vi "OrderNotclose.vi"(8 "错误输入（无错误）":errorcluster, 9 "关闭通道":u16(ring) items=["CH1", "CH2", "CH3", "CH4"], 10 "打开通道":u16(ring) items=["CH1", "CH2", "CH3", "CH4"], 11 "VISA资源名称":refnum<visa-resource-name>="DPO5054-C012667") -> (0 "错误输出":errorcluster, 2 "输出数组":dbl[](array[numeric]), 3 "VISA资源名称 2":refnum<visa-resource-name>)   [LabVIEW 2014]
panel:
  out "AMP":dbl
  out "RMS":dbl
  out "MAX":dbl
  out "MIN":dbl
  out "PK2PK":dbl
  out "PERIOD":dbl
  out "FREQ":dbl
  out "RISETIME":dbl
  out "FallTime":dbl
  out "PosWidth":dbl
  out "NegWidth":dbl
  out "PositiveDutyCycle":dbl
  out "NegativeDutyCycle":dbl
  out "ACRMS":dbl
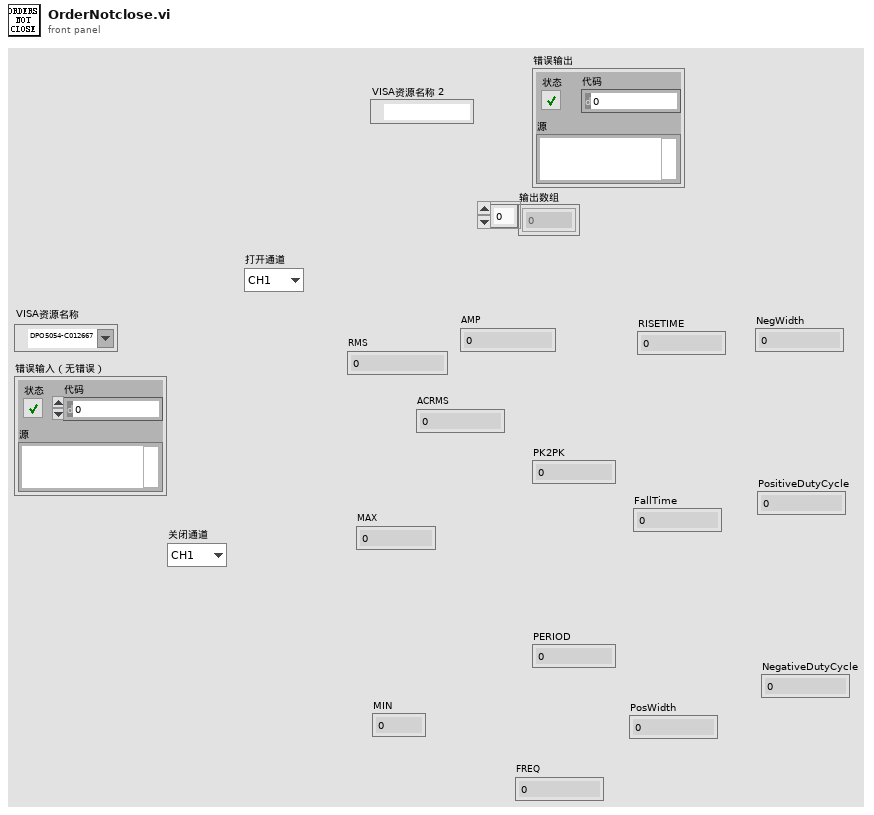
[diagram p1: front panel]
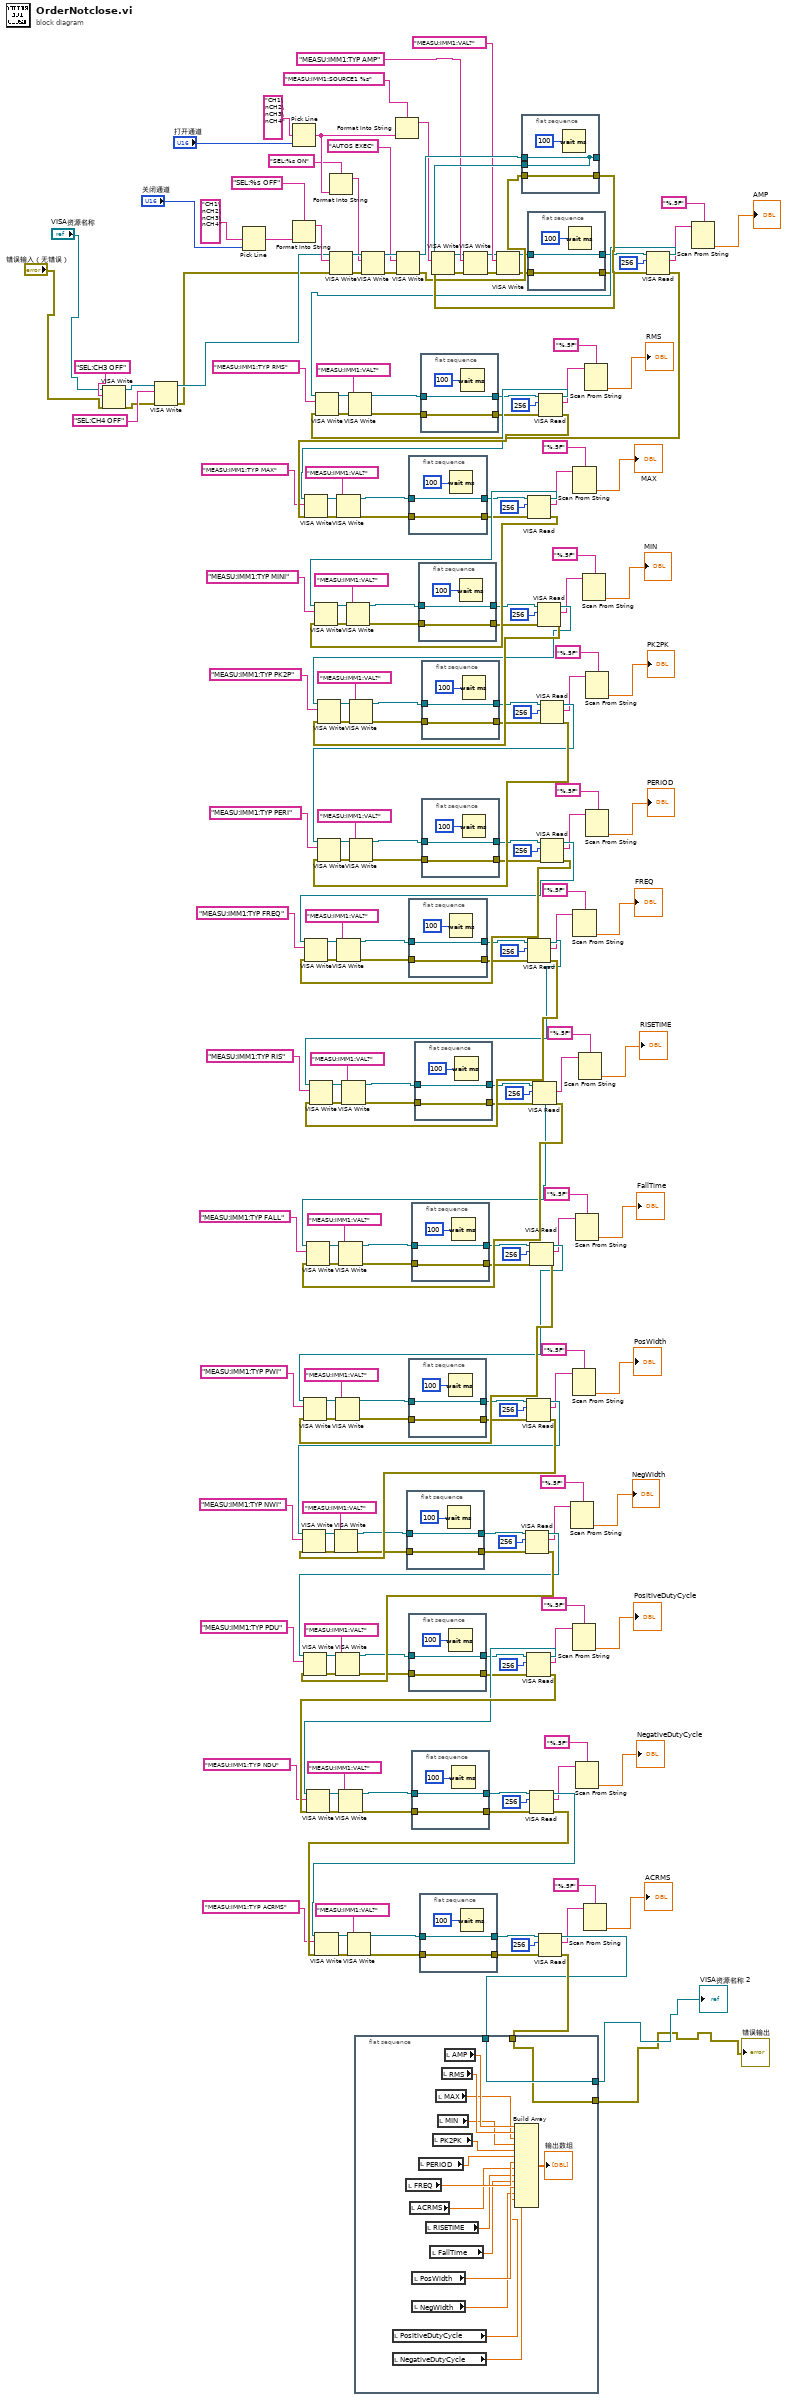
[diagram p0: block diagram]
diagram:
  n1 = VISA Write(VISA resource name="VISA资源名称", write buffer="SEL:CH3 OFF" ("格式字符串"), error in (no error)="错误输入（无错误）") -> (VISA resource name out=w6:refnum<visa-resource-name>, error out=w7:errorcluster)  [unwired: 1 out]
  n2 = VISA Write(VISA resource name=w6, write buffer="SEL:CH4 OFF" ("格式字符串"), error in (no error)=w7) -> (VISA resource name out=w2:refnum<visa-resource-name>, error out=w1:errorcluster)  [unwired: 1 out]
  n3 = Pick Line(multi-line string="CH1\nCH2\nCH3\nCH4" ("多行字符串"), line index="关闭通道") -> (output string=w30:string)  [unwired: 1 in]
  n4 = Pick Line(multi-line string="CH1\nCH2\nCH3\nCH4" ("多行字符串"), line index="打开通道") -> (output string=w25:string)  [unwired: 1 in]
  n5 = Format Into String(format string="SEL:%s OFF" ("格式字符串"), w30) -> (resulting string=w34:string)  [unwired: 2 in, 1 out]
  n6 = Format Into String(format string="SEL:%s ON" ("格式字符串"), w25) -> (resulting string=w26:string)  [unwired: 2 in, 1 out]
  n7 = VISA Write(VISA resource name=w2, write buffer=w34, error in (no error)=w1) -> (VISA resource name out=w35:refnum<visa-resource-name>, error out=w36:errorcluster)  [unwired: 1 out]
  n8 = flat-sequence {
    tunnel: w227 -> [w231]
    tunnel: [w231] -> w229
    tunnel: w228 -> [w230]
    tunnel: [w230] -> w9
    frame #0 {
      n9 = local read "PositiveDutyCycle"() -> (w234:dbl)
      n10 = local read "NegativeDutyCycle"() -> (w233:dbl)
      n11 = local read "FREQ"() -> (w240:dbl)
      n12 = local read "ACRMS"() -> (w239:dbl)
      n13 = local read "PosWidth"() -> (w236:dbl)
      n14 = local read "NegWidth"() -> (w235:dbl)
      n15 = local read "PERIOD"() -> (w241:dbl)
      n16 = local read "RISETIME"() -> (w238:dbl)
      n17 = local read "FallTime"() -> (w237:dbl)
      n18 = local read "PK2PK"() -> (w242:dbl)
      n19 = local read "MAX"() -> (w244:dbl)
      n20 = local read "MIN"() -> (w243:dbl)
      n21 = local read "RMS"() -> (w245:dbl)
      n22 = local read "AMP"() -> (w246:dbl)
      n23 = Build Array(w246, w245, w244, w243, w242, w241, w240, w239, w238, w237, w236, w235, w234, w233) -> (→"输出数组":dbl[])
    }
  }
  n24 = VISA Write(VISA resource name=w35, write buffer=w26, error in (no error)=w36) -> (VISA resource name out=w28:refnum<visa-resource-name>, error out=w29:errorcluster)  [unwired: 1 out]
  n25 = Format Into String(format string="MEASU:IMM1:SOURCE1 %s" ("格式字符串"), w25) -> (resulting string=w12:string)  [unwired: 2 in, 1 out]
  n26 = VISA Write(VISA resource name=w28, write buffer="AUTOS EXEC" ("写入缓冲区"), error in (no error)=w29) -> (VISA resource name out=w125:refnum<visa-resource-name>, error out=w126:errorcluster)  [unwired: 1 out]
  n27 = flat-sequence {
    tunnel: w166 -> [w248]
    tunnel: [w248] -> w168
    tunnel: w165 -> [w247]
    tunnel: [w247] -> w169
    frame #0 {
      n28 = Wait (ms)(milliseconds to wait=u32 100 ("等待时间（毫秒）")) -> ()  [unwired: 1 out]
    }
  }
  n29 = flat-sequence {
    tunnel: w163 -> [w251]
    tunnel: [w251] -> w161
    tunnel: w164 -> [w250]
    tunnel: [w250] -> w160
    frame #0 {
      n30 = Wait (ms)(milliseconds to wait=u32 100 ("等待时间（毫秒）")) -> ()  [unwired: 1 out]
    }
  }
  n31 = flat-sequence {
    tunnel: w187 -> [w254]
    tunnel: [w254] -> w185
    tunnel: w188 -> [w253]
    tunnel: [w253] -> w184
    frame #0 {
      n32 = Wait (ms)(milliseconds to wait=u32 100 ("等待时间（毫秒）")) -> ()  [unwired: 1 out]
    }
  }
  n33 = flat-sequence {
    tunnel: w54 -> [w257]
    tunnel: [w257] -> w56
    tunnel: w53 -> [w256]
    tunnel: [w256] -> w57
    frame #0 {
      n34 = Wait (ms)(milliseconds to wait=u32 100 ("等待时间（毫秒）")) -> ()  [unwired: 1 out]
    }
  }
  n35 = flat-sequence {
    tunnel: w102 -> [w260]
    tunnel: [w260] -> w104
    tunnel: w101 -> [w259]
    tunnel: [w259] -> w105
    frame #0 {
      n36 = Wait (ms)(milliseconds to wait=u32 100 ("等待时间（毫秒）")) -> ()  [unwired: 1 out]
    }
  }
  n37 = flat-sequence {
    tunnel: w142 -> [w263]
    tunnel: [w263] -> w144
    tunnel: w141 -> [w262]
    tunnel: [w262] -> w145
    frame #0 {
      n38 = Wait (ms)(milliseconds to wait=u32 100 ("等待时间（毫秒）")) -> ()  [unwired: 1 out]
    }
  }
  n39 = flat-sequence {
    tunnel: w190 -> [w266]
    tunnel: [w266] -> w192
    tunnel: w189 -> [w265]
    tunnel: [w265] -> w193
    frame #0 {
      n40 = Wait (ms)(milliseconds to wait=u32 100 ("等待时间（毫秒）")) -> ()  [unwired: 1 out]
    }
  }
  n41 = flat-sequence {
    tunnel: w139 -> [w269]
    tunnel: [w269] -> w137
    tunnel: w140 -> [w268]
    tunnel: [w268] -> w136
    frame #0 {
      n42 = Wait (ms)(milliseconds to wait=u32 100 ("等待时间（毫秒）")) -> ()  [unwired: 1 out]
    }
  }
  n43 = flat-sequence {
    tunnel: w75 -> [w272]
    tunnel: [w272] -> w73
    tunnel: w76 -> [w271]
    tunnel: [w271] -> w72
    frame #0 {
      n44 = Wait (ms)(milliseconds to wait=u32 100 ("等待时间（毫秒）")) -> ()  [unwired: 1 out]
    }
  }
  n45 = flat-sequence {
    tunnel: w223 -> [w275]
    tunnel: [w275] -> w221
    tunnel: w224 -> [w274]
    tunnel: [w274] -> w220
    frame #0 {
      n46 = Wait (ms)(milliseconds to wait=u32 100 ("等待时间（毫秒）")) -> ()  [unwired: 1 out]
    }
  }
  n47 = flat-sequence {
    tunnel: w51 -> [w278]
    tunnel: [w278] -> w49
    tunnel: w52 -> [w277]
    tunnel: [w277] -> w48
    frame #0 {
      n48 = Wait (ms)(milliseconds to wait=u32 100 ("等待时间（毫秒）")) -> ()  [unwired: 1 out]
    }
  }
  n49 = flat-sequence {
    tunnel: w78 -> [w281]
    tunnel: [w281] -> w80
    tunnel: w77 -> [w280]
    tunnel: [w280] -> w81
    frame #0 {
      n50 = Wait (ms)(milliseconds to wait=u32 100 ("等待时间（毫秒）")) -> ()  [unwired: 1 out]
    }
  }
  n51 = flat-sequence {
    tunnel: w99 -> [w284]
    tunnel: [w284] -> w97
    tunnel: w100 -> [w283]
    tunnel: [w283] -> w96
    frame #0 {
      n52 = Wait (ms)(milliseconds to wait=u32 100 ("等待时间（毫秒）")) -> ()  [unwired: 1 out]
    }
  }
  n53 = VISA Write(VISA resource name=w127, write buffer=w12, error in (no error)=w128) -> (VISA resource name out=w15:refnum<visa-resource-name>, error out=w16:errorcluster)  [unwired: 1 out]
  n54 = VISA Write(VISA resource name=w15, write buffer="MEASU:IMM1:TYP AMP" ("写入缓冲区"), error in (no error)=w16) -> (VISA resource name out=w19:refnum<visa-resource-name>, error out=w20:errorcluster)  [unwired: 1 out]
  n55 = VISA Write(VISA resource name=w19, write buffer="MEASU:IMM1:VAL?" ("写入缓冲区"), error in (no error)=w20) -> (VISA resource name out=w22:refnum<visa-resource-name>, error out=w23:errorcluster)  [unwired: 1 out]
  n56 = flat-sequence {
    tunnel: w125 -> [w286]
    tunnel: [w286] -> _
    tunnel: w126 -> [w287]
    tunnel: [w287] -> w128
    tunnel: [w286] -> w127
    frame #0 {
      n57 = Wait (ms)(milliseconds to wait=u32 100 ("等待时间（毫秒）")) -> ()  [unwired: 1 out]
    }
  }
  n58 = VISA Read(VISA resource name=w168, byte count=u32 256 ("字节总数"), error in (no error)=w169) -> (VISA resource name out=w209:refnum<visa-resource-name>, read buffer=w170:string, error out=w210:errorcluster)  [unwired: 1 out]
  n59 = VISA Write(VISA resource name=w209, write buffer="MEASU:IMM1:TYP PDU" ("写入缓冲区"), error in (no error)=w210) -> (VISA resource name out=w179:refnum<visa-resource-name>, error out=w178:errorcluster)  [unwired: 1 out]
  n60 = VISA Write(VISA resource name=w179, write buffer="MEASU:IMM1:VAL?" ("写入缓冲区"), error in (no error)=w178) -> (VISA resource name out=w187:refnum<visa-resource-name>, error out=w188:errorcluster)  [unwired: 1 out]
  n61 = VISA Read(VISA resource name=w161, byte count=u32 256 ("字节总数"), error in (no error)=w160) -> (VISA resource name out=w207:refnum<visa-resource-name>, read buffer=w159:string, error out=w208:errorcluster)  [unwired: 1 out]
  n62 = VISA Write(VISA resource name=w207, write buffer="MEASU:IMM1:TYP NWI" ("写入缓冲区"), error in (no error)=w208) -> (VISA resource name out=w174:refnum<visa-resource-name>, error out=w175:errorcluster)  [unwired: 1 out]
  n63 = VISA Write(VISA resource name=w174, write buffer="MEASU:IMM1:VAL?" ("写入缓冲区"), error in (no error)=w175) -> (VISA resource name out=w166:refnum<visa-resource-name>, error out=w165:errorcluster)  [unwired: 1 out]
  n64 = VISA Read(VISA resource name=w185, byte count=u32 256 ("字节总数"), error in (no error)=w184) -> (VISA resource name out=w211:refnum<visa-resource-name>, read buffer=w183:string, error out=w212:errorcluster)  [unwired: 1 out]
  n65 = VISA Write(VISA resource name=w211, write buffer="MEASU:IMM1:TYP NDU" ("写入缓冲区"), error in (no error)=w212) -> (VISA resource name out=w198:refnum<visa-resource-name>, error out=w199:errorcluster)  [unwired: 1 out]
  n66 = VISA Write(VISA resource name=w198, write buffer="MEASU:IMM1:VAL?" ("写入缓冲区"), error in (no error)=w199) -> (VISA resource name out=w190:refnum<visa-resource-name>, error out=w189:errorcluster)  [unwired: 1 out]
  n67 = flat-sequence {
    tunnel: w22 -> [w290]
    tunnel: [w290] -> w17
    tunnel: w23 -> [w289]
    tunnel: [w289] -> w18
    frame #0 {
      n68 = Wait (ms)(milliseconds to wait=u32 100 ("等待时间（毫秒）")) -> ()  [unwired: 1 out]
    }
  }
  n69 = VISA Read(VISA resource name=w56, byte count=u32 256 ("字节总数"), error in (no error)=w57) -> (VISA resource name out=w117:refnum<visa-resource-name>, read buffer=w58:string, error out=w118:errorcluster)  [unwired: 1 out]
  n70 = VISA Write(VISA resource name=w117, write buffer="MEASU:IMM1:TYP MINI" ("写入缓冲区"), error in (no error)=w118) -> (VISA resource name out=w67:refnum<visa-resource-name>, error out=w66:errorcluster)  [unwired: 1 out]
  n71 = VISA Write(VISA resource name=w67, write buffer="MEASU:IMM1:VAL?" ("写入缓冲区"), error in (no error)=w66) -> (VISA resource name out=w75:refnum<visa-resource-name>, error out=w76:errorcluster)  [unwired: 1 out]
  n72 = VISA Read(VISA resource name=w104, byte count=u32 256 ("字节总数"), error in (no error)=w105) -> (VISA resource name out=w201:refnum<visa-resource-name>, read buffer=w106:string, error out=w202:errorcluster)  [unwired: 1 out]
  n73 = VISA Write(VISA resource name=w201, write buffer="MEASU:IMM1:TYP RIS" ("写入缓冲区"), error in (no error)=w202) -> (VISA resource name out=w131:refnum<visa-resource-name>, error out=w130:errorcluster)  [unwired: 1 out]
  n74 = VISA Write(VISA resource name=w131, write buffer="MEASU:IMM1:VAL?" ("写入缓冲区"), error in (no error)=w130) -> (VISA resource name out=w139:refnum<visa-resource-name>, error out=w140:errorcluster)  [unwired: 1 out]
  n75 = VISA Read(VISA resource name=w144, byte count=u32 256 ("字节总数"), error in (no error)=w145) -> (VISA resource name out=w205:refnum<visa-resource-name>, read buffer=w146:string, error out=w206:errorcluster)  [unwired: 1 out]
  n76 = VISA Write(VISA resource name=w205, write buffer="MEASU:IMM1:TYP PWI" ("写入缓冲区"), error in (no error)=w206) -> (VISA resource name out=w155:refnum<visa-resource-name>, error out=w154:errorcluster)  [unwired: 1 out]
  n77 = VISA Write(VISA resource name=w155, write buffer="MEASU:IMM1:VAL?" ("写入缓冲区"), error in (no error)=w154) -> (VISA resource name out=w163:refnum<visa-resource-name>, error out=w164:errorcluster)  [unwired: 1 out]
  n78 = VISA Read(VISA resource name=w192, byte count=u32 256 ("字节总数"), error in (no error)=w193) -> (VISA resource name out=w225:refnum<visa-resource-name>, read buffer=w194:string, error out=w226:errorcluster)  [unwired: 1 out]
  n79 = VISA Write(VISA resource name=w225, write buffer="MEASU:IMM1:TYP ACRMS" ("写入缓冲区"), error in (no error)=w226) -> (VISA resource name out=w215:refnum<visa-resource-name>, error out=w214:errorcluster)  [unwired: 1 out]
  n80 = VISA Write(VISA resource name=w215, write buffer="MEASU:IMM1:VAL?" ("写入缓冲区"), error in (no error)=w214) -> (VISA resource name out=w223:refnum<visa-resource-name>, error out=w224:errorcluster)  [unwired: 1 out]
  n81 = VISA Read(VISA resource name=w137, byte count=u32 256 ("字节总数"), error in (no error)=w136) -> (VISA resource name out=w203:refnum<visa-resource-name>, read buffer=w135:string, error out=w204:errorcluster)  [unwired: 1 out]
  n82 = VISA Write(VISA resource name=w203, write buffer="MEASU:IMM1:TYP FALL" ("写入缓冲区"), error in (no error)=w204) -> (VISA resource name out=w150:refnum<visa-resource-name>, error out=w151:errorcluster)  [unwired: 1 out]
  n83 = VISA Write(VISA resource name=w150, write buffer="MEASU:IMM1:VAL?" ("写入缓冲区"), error in (no error)=w151) -> (VISA resource name out=w142:refnum<visa-resource-name>, error out=w141:errorcluster)  [unwired: 1 out]
  n84 = VISA Read(VISA resource name=w73, byte count=u32 256 ("字节总数"), error in (no error)=w72) -> (VISA resource name out=w119:refnum<visa-resource-name>, read buffer=w71:string, error out=w120:errorcluster)  [unwired: 1 out]
  n85 = VISA Write(VISA resource name=w119, write buffer="MEASU:IMM1:TYP PK2P" ("写入缓冲区"), error in (no error)=w120) -> (VISA resource name out=w86:refnum<visa-resource-name>, error out=w87:errorcluster)  [unwired: 1 out]
  n86 = VISA Write(VISA resource name=w86, write buffer="MEASU:IMM1:VAL?" ("写入缓冲区"), error in (no error)=w87) -> (VISA resource name out=w78:refnum<visa-resource-name>, error out=w77:errorcluster)  [unwired: 1 out]
  n87 = VISA Read(VISA resource name=w221, byte count=u32 256 ("字节总数"), error in (no error)=w220) -> (VISA resource name out=w227:refnum<visa-resource-name>, read buffer=w219:string, error out=w228:errorcluster)  [unwired: 1 out]
  n88 = VISA Read(VISA resource name=w49, byte count=u32 256 ("字节总数"), error in (no error)=w48) -> (VISA resource name out=w115:refnum<visa-resource-name>, read buffer=w47:string, error out=w116:errorcluster)  [unwired: 1 out]
  n89 = VISA Write(VISA resource name=w115, write buffer="MEASU:IMM1:TYP MAX" ("写入缓冲区"), error in (no error)=w116) -> (VISA resource name out=w62:refnum<visa-resource-name>, error out=w63:errorcluster)  [unwired: 1 out]
  n90 = VISA Write(VISA resource name=w62, write buffer="MEASU:IMM1:VAL?" ("写入缓冲区"), error in (no error)=w63) -> (VISA resource name out=w54:refnum<visa-resource-name>, error out=w53:errorcluster)  [unwired: 1 out]
  n91 = VISA Read(VISA resource name=w80, byte count=u32 256 ("字节总数"), error in (no error)=w81) -> (VISA resource name out=w121:refnum<visa-resource-name>, read buffer=w82:string, error out=w122:errorcluster)  [unwired: 1 out]
  n92 = VISA Write(VISA resource name=w121, write buffer="MEASU:IMM1:TYP PERI" ("写入缓冲区"), error in (no error)=w122) -> (VISA resource name out=w91:refnum<visa-resource-name>, error out=w90:errorcluster)  [unwired: 1 out]
  n93 = VISA Write(VISA resource name=w91, write buffer="MEASU:IMM1:VAL?" ("写入缓冲区"), error in (no error)=w90) -> (VISA resource name out=w99:refnum<visa-resource-name>, error out=w100:errorcluster)  [unwired: 1 out]
  n94 = VISA Read(VISA resource name=w97, byte count=u32 256 ("字节总数"), error in (no error)=w96) -> (VISA resource name out=w123:refnum<visa-resource-name>, read buffer=w95:string, error out=w124:errorcluster)  [unwired: 1 out]
  n95 = VISA Write(VISA resource name=w123, write buffer="MEASU:IMM1:TYP FREQ" ("写入缓冲区"), error in (no error)=w124) -> (VISA resource name out=w110:refnum<visa-resource-name>, error out=w111:errorcluster)  [unwired: 1 out]
  n96 = VISA Write(VISA resource name=w110, write buffer="MEASU:IMM1:VAL?" ("写入缓冲区"), error in (no error)=w111) -> (VISA resource name out=w102:refnum<visa-resource-name>, error out=w101:errorcluster)  [unwired: 1 out]
  n97 = Scan From String(format string="%.5F" ("格式字符串"), input string=w170) -> (output 1=→"NegWidth":dbl)  [unwired: 3 in, 3 out]
  n98 = Scan From String(format string="%.5F" ("格式字符串"), input string=w159) -> (output 1=→"PosWidth":dbl)  [unwired: 3 in, 3 out]
  n99 = Scan From String(format string="%.5F" ("格式字符串"), input string=w183) -> (output 1=→"PositiveDutyCycle":dbl)  [unwired: 3 in, 3 out]
  n100 = Scan From String(format string="%.5F" ("格式字符串"), input string=w58) -> (output 1=→"MAX":dbl)  [unwired: 3 in, 3 out]
  n101 = Scan From String(format string="%.5F" ("格式字符串"), input string=w106) -> (output 1=→"FREQ":dbl)  [unwired: 3 in, 3 out]
  n102 = Scan From String(format string="%.5F" ("格式字符串"), input string=w146) -> (output 1=→"FallTime":dbl)  [unwired: 3 in, 3 out]
  n103 = Scan From String(format string="%.5F" ("格式字符串"), input string=w194) -> (output 1=→"NegativeDutyCycle":dbl)  [unwired: 3 in, 3 out]
  n104 = Scan From String(format string="%.5F" ("格式字符串"), input string=w135) -> (output 1=→"RISETIME":dbl)  [unwired: 3 in, 3 out]
  n105 = Scan From String(format string="%.5F" ("格式字符串"), input string=w71) -> (output 1=→"MIN":dbl)  [unwired: 3 in, 3 out]
  n106 = Scan From String(format string="%.5F" ("格式字符串"), input string=w219) -> (output 1=→"ACRMS":dbl)  [unwired: 3 in, 3 out]
  n107 = Scan From String(format string="%.5F" ("格式字符串"), input string=w47) -> (output 1=→"RMS":dbl)  [unwired: 3 in, 3 out]
  n108 = Scan From String(format string="%.5F" ("格式字符串"), input string=w82) -> (output 1=→"PK2PK":dbl)  [unwired: 3 in, 3 out]
  n109 = Scan From String(format string="%.5F" ("格式字符串"), input string=w95) -> (output 1=→"PERIOD":dbl)  [unwired: 3 in, 3 out]
  n110 = VISA Read(VISA resource name=w17, byte count=u32 256 ("字节总数"), error in (no error)=w18) -> (VISA resource name out=w113:refnum<visa-resource-name>, read buffer=w38:string, error out=w114:errorcluster)  [unwired: 1 out]
  n111 = VISA Write(VISA resource name=w113, write buffer="MEASU:IMM1:TYP RMS" ("写入缓冲区"), error in (no error)=w114) -> (VISA resource name out=w43:refnum<visa-resource-name>, error out=w42:errorcluster)  [unwired: 1 out]
  n112 = VISA Write(VISA resource name=w43, write buffer="MEASU:IMM1:VAL?" ("写入缓冲区"), error in (no error)=w42) -> (VISA resource name out=w51:refnum<visa-resource-name>, error out=w52:errorcluster)  [unwired: 1 out]
  n113 = Scan From String(format string="%.5F" ("格式字符串"), input string=w38) -> (output 1=→"AMP":dbl)  [unwired: 3 in, 3 out]
  "错误输出" <- w9
  "VISA资源名称 2" <- w229
